vi "Load Custom Status Glyph.vi"(7 "tree ref":refnum<vi>, 8 "error in":errorcluster, 11 "glyph directories":path[](array[path])) -> (0 "error out":errorcluster)   [LabVIEW 2013, in "configuration library.lvlib"]
uses:
  configuration library.lvlib
  <vilib>/CEF_TreeControl/Controls/GlyphIndexPair.ctl
  <vilib>/CEF_TreeControl/Controls/GlyphIndexPairActions.ctl
  Configuration Editor/subVIs/Glyphs Status.ctl
  <vilib>/CEF_TreeControl/NISE_CEF_TreeControl.lvlib
  Configuration Editor/PL Framework Configuration Tool.lvlib
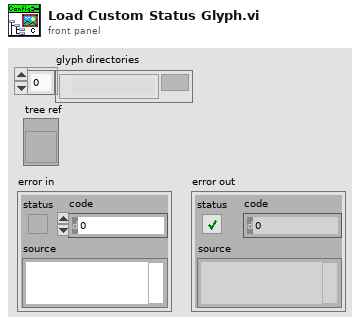
[diagram p1: front panel]
types:
  T1 = typedef "PL Framework Configuration Tool.lvlib/Glyphs Status.ctl" = enum16{"Normal", "Error", "Async"}
  T2 = typedef "NISE_CEF_TreeControl.lvlib/GlyphIndexPairActions.ctl" = enum16{"Get", "Initialize"}
  T3 = typedef "NISE_CEF_TreeControl.lvlib/GlyphIndexPair.ctl" = cluster{"name":string, "index":i32}
  T4 = typedef "imagedata.ctl" = cluster{"image type":i32, "image depth":i32, "image":u8[], "mask":u8[], "colors":u32[], "Rectangle":cluster{"left":i16, "top":i16, "right":i16, "bottom":i16}}
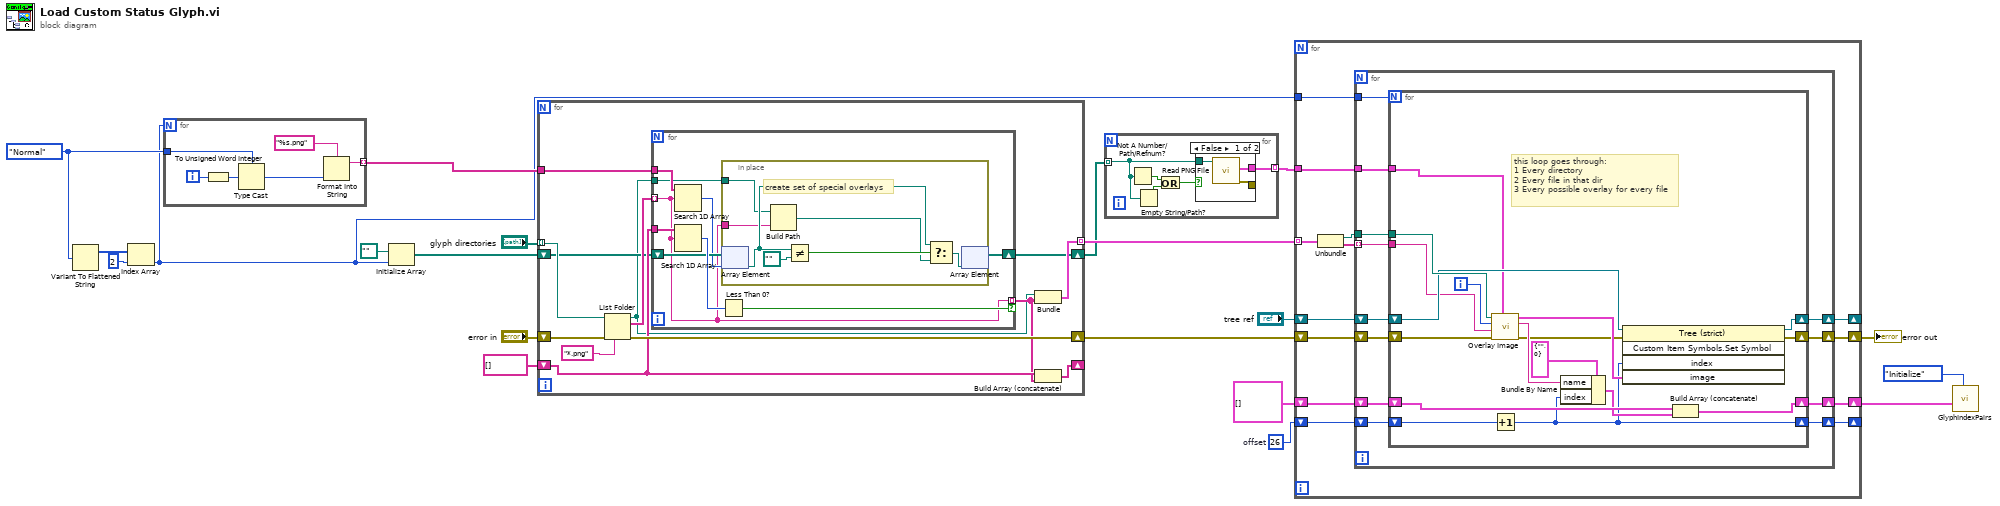
[diagram p0: block diagram]
diagram:
  w5 = Glyphs_Status."Normal" ("Enum")
  w13 = 26  # offset
  n1 = Variant To Flattened String(Variant=w5) -> (1:w9:i16[])  [unwired: 1 out]
  n2 = Index Array(array=w9, index=2) -> (element=w3:i16)
  n3 = for {
    N: w3 -> [_]
    tunnel: w5 -> [w24]
    tunnel: [w21] -> w4 mode=indexing
    i -> [w26]
    n4 = To Unsigned Word Integer(number=w26) -> (unsigned 16bit integer=w25:u16)
    n5 = Type Cast(type=w24, x=w25) -> (*(type *) &x=w23:T1)
    n6 = Format Into String(format string="%s.png", w23) -> (resulting string=w21:string)  [unwired: 2 in, 1 out]
  }
  n7 = Initialize Array(path "", w3) -> (w6:path[])
  n8 = for {
    tunnel: "glyph directories" -> [w39] mode=indexing
    tunnel: [w35] -> w11 mode=indexing
    shift-right: [w36] -> w12
    shift-left: "error in" -> [w38]
    shift-right: [w34] -> _
    shift-left: string[] [] -> [w32]
    shift-right: [w28] -> w2
    shift-left: w6 -> [w29]
    tunnel: w4 -> [w30]
    n9 = List Folder(path=w39, pattern="*.png", error in=w38) -> (path out=w27:path, filenames=w33:string[], error out=w36:errorcluster)  [unwired: 1 in, 1 out]
    n10 = for {
      tunnel: w33 -> [w40] mode=indexing
      tunnel: w32 -> [w48]
      tunnel: [w40] -> w31 mode=indexing if=w46
      tunnel: w30 -> [w45]
      shift-right: [w43] -> w28
      shift-left: w29 -> [w44]
      tunnel: w27 -> [w41]
      n11 = Search 1D Array(1D array=w45, element=w40) -> (index of element=w42:i32)  [unwired: 1 in]
      n12 = Search 1D Array(1D array=w48, element=w40) -> (index of element=w47:i32)  [unwired: 1 in]
      n13 = Less Than 0?(x=w47) -> (x < 0?=w46:bool)
      n14 = in-place {
        in-place-border: w41 -> [w50]
        in-place-border: w40 -> [w49]
        # "create set of special overlays"
        n15 = in-place-array #1(w44, w42) -> (w53:path)
        n16 = Build Path(base path=w50, name or relative path=w49) -> (appended path=w51:path)
        n17 = Not Equal?(x=w53, y=path "") -> (x != y?=w54:bool)
        n18 = Select(t=w53, s=w54, f=w51) -> (s? t:f=w52:path)
        n19 = in-place-array #1(w52) -> (w43:path[])  [unwired: 1 out]
      }
    }
    n20 = Bundle("path out"=w27, w31) -> (w35:cluster{"path out":path, string[]})  [unwired: 1 in]
    n21 = Build Array (concatenate)(w32, w31) -> (w34:string[])
  }
  n22 = for {
    tunnel: w2 -> [w56] mode=indexing
    tunnel: [w60] -> w1 mode=indexing
    n23 = Not A Number/Path/Refnum?(number/path/refnum=w56) -> (NaN/Path/Refnum?=w58:bool)
    n24 = Empty String/Path?(string/path=w56) -> (empty?=w57:bool)
    n25 = Or(x=w58, y=w57) -> (x .or. y?=w59:bool)
    n26 = case shown="False" w59 {
      tunnel: w56 -> [w63 _]
      tunnel: [w62 _] -> w60
      tunnel: [w61 _] -> _
      frame False {
        n27 = call <vilib>:"Read PNG File.vi"("path to PNG file"=w63) -> ("error out"=w61:errorcluster, "image data"=w62:T4)  [unwired: 8 in, 1 out]
      }
      frame True {
      }
    }
  }
  n28 = for {
    shift-right: [w72] -> w16
    shift-left: T3[] [] ("array") -> [w73]
    shift-right: [w71] -> _
    shift-left: "tree ref" -> [w76]
    shift-right: [w69] -> _
    shift-left: w13 -> [w70]
    shift-right: [w74] -> w14
    shift-left: w12 -> [w75]
    tunnel: w11 -> [w68] mode=indexing
    tunnel: w3 -> [w65]
    tunnel: w1 -> [w64]
    n29 = Unbundle(w68) -> ("path out"=w67:path, w66:string[])
    n30 = for {
      tunnel: w67 -> [w80]
      tunnel: w66 -> [w79] mode=indexing
      shift-right: [w84] -> w72
      shift-left: w73 -> [w85]
      shift-right: [w81] -> w69
      shift-left: w70 -> [w82]
      shift-right: [w83] -> w71
      shift-left: w76 -> [w88]
      shift-right: [w86] -> w74
      shift-left: w75 -> [w87]
      tunnel: w65 -> [w78]
      tunnel: w64 -> [w77]
      n31 = for {
        N: w78 -> [_]
        tunnel: w80 -> [w105]
        tunnel: w79 -> [w100]
        shift-right: [w103] -> w83
        shift-left: w88 -> [w104]
        shift-right: [w98] -> w86
        shift-left: w87 -> [w94]
        shift-right: [w96] -> w84
        shift-left: w85 -> [w101]
        shift-right: [w90] -> w81
        shift-left: w82 -> [w91]
        tunnel: w77 -> [w89]
        i -> [w92]
        # "this loop goes through:\n1 Every directory\n2 Every file in that dir\n3 Every possible overlay for every file"
        n32 = call "Overlay Image.vi"("overlay images"=w89, "error in"=w94, "image name in"=w100, "overlay"=w92, "path in"=w105) -> ("error out"=w93:errorcluster, "overlayed image name"=w95:string, "image data"=w102:T4)  [unwired: 4 in]
        n33 = Increment(x=w91) -> (x+1=w90:i32)
        n34 = Bundle By Name(cluster=T3 {"name"="", "index"=0} ("glyphIndexPair"), "name"=w95, "index"=w90) -> (w99:T3)
        n35 = invoke class="Tree (strict)" method="Custom Item Symbols.Set Symbol"(reference=w104, error in=w93, "index"=w90, "image"=w102) -> (reference out=w103:refnum<vi>, error out=w98:errorcluster)  [unwired: 1 in, 3 out]
        n36 = Build Array (concatenate)(w101, w99) -> (w96:T3[])
      }
    }
  }
  "error out" <- w14
  n37 = call <vilib>:"GlyphIndexPairs.vi"("enum"=GlyphIndexPairActions."Initialize" ("Enum"), "array"=w16) -> ()  [unwired: 9 in, 1 out]
